vi "Process.vi"(8 "error in":errorcluster, 11 "Plugin in":refnum<class "DFT_Spectra.lvclass">) -> (0 "error out":errorcluster, 3 "Plugin out":refnum<class "DFT_Spectra.lvclass">)   [LabVIEW 2024, in "DFT_Spectra.lvlib" / "DFT_Spectra.lvclass"]
uses:
  DFT_Spectra.lvclass
  DFT_Spectra.lvclass/DFT_Spectra.ctl
  <vilib>/addons/_NISVFA/_Shared subVIs/Data Objects/Waveforms (DBL)/SV Read Next Overlapping Data.vi
  <vilib>/FlexLogger/SDK/PluginSDK.lvlibp/PEFClasses/SDK/Plugin/Plugin.lvclass
  <vilib>/addons/_NISVFA/_Shared subVIs/Data Objects/Waveforms (DBL)/Waveforms (N Ch).lvclass
  C:/Program Files/National Instruments/LabVIEW 2024/vi.lib/FlexLogger/SDK/PluginSDK.lvlibp/PEFClasses/SDK/Plugin/Plugin.lvclass
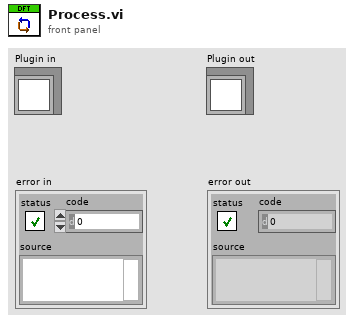
[diagram p1: front panel]
types:
  T1 = typedef "DFT_Spectra.lvlib/DFT_Spectra.lvclass/DFT_Spectra Data.ctl" = cluster{"First Time":bool, "Show Results Window":bool, "Show Results Window Clicked":bool, "Window":T2, "overlap":i32, "Block Duration":dbl, "Averaging parameters":cluster{"averaging mode":enum16{"No averaging", "Vector averaging", "RMS averaging", "Peak hold"}, "weighting mode":enum16{"Linear", "Exponential"}, "number of averages":u32}, "buffer out":refnum<data-value>, "Avg Spectra":refnum<vi>, "Spectra UI":refnum<vi>}
  T2 = typedef "NI_AALPro.lvlib/windowTd.ctl" = u32
  T3 = typedef "svc_Spectrum Info.ctl" = cluster{"channel name":string, "description":string, "x-axis units":T4, "spectral info":cluster{"spectrum type":T5, "linear/dB":enum16{"linear", "dB"}, "window":u16, "window size":i32, "FFT size":i32}, "engineering units":T6, "custom label":string, "dB reference [EU]":dbl, "peak units":enum16{"rms", "peak", "peak-peak"}, "weighting filter":T7, "spectral density?":bool, "unit label":string, "spectrum skewed?":bool, "complimentary spectrum units":T8}
  T4 = typedef "svc_X-Axis Units.ctl" = u16
  T5 = typedef "svc_Spectrum Type.ctl" = enum16{"FFT Spectrum [complex]", "Amplitude [Magnitude]", "Power [Magnitude^2]", "Cross Spectrum [complex]", "Frequency Response [Complex]"}
  T6 = typedef "svc_Engineering Units Text Ring.ctl" = u16
  T7 = typedef "svc_Weighting Filter Text Ring.ctl" = u16
  T8 = typedef "svc_Complimentary Spectrum Units.ctl" = enum16{"none", "radians", "degrees", "cycles", "imaginary"}
  T9 = cluster{"power spectra":cluster{"f0":dbl, "df":dbl, "magnitude":dbl[]}[], "spectra info":T3[], "data valid":bool, "averages completed":dbl}
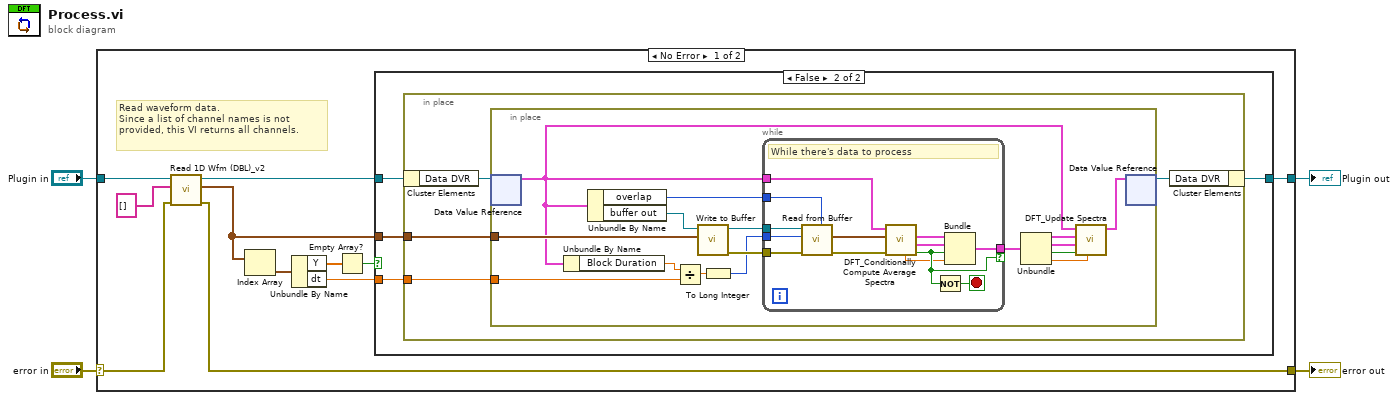
[diagram p0: block diagram]
diagram:
  n1 = case shown="No Error" "error in" {
    selector: "error in" -> [w14 w54]
    tunnel: [w13 w55] -> w3
    tunnel: "Plugin in" -> [w15 w55]
    tunnel: [w5 w54] -> w2
    frame No Error {
      # "Read waveform data.\nSince a list of channel names is not provided, this VI returns all channels."
      n2 = call <vilib>:"Read 1D Wfm (DBL)_v2.vi"("error in (no error)"=w14, "Unique Identifers (empty = all)"=string[] [] ("Unique Channel Identifers (empty = all)"), "Plugin in"=w15) -> ("error out"=w5:errorcluster, "Data"=w10:waveform(dbl)[], "Plugin out"=w12:refnum<class "DFT_Spectra.lvclass">)  [unwired: 5 in, 1 out]
      n3 = Index Array(array=w10) -> (element=w9:waveform(dbl))  [unwired: 1 in]
      n4 = Unbundle By Name(w9) -> ("Y"=w8:dbl[], "dt"=w6:dbl)
      n5 = Empty Array?(array=w8) -> (empty?=w7:bool)
      n6 = case shown="False" w7 {
        tunnel: w10 -> [_ w20]
        tunnel: [w16 w17] -> w13
        tunnel: w12 -> [w16 w18]
        tunnel: w6 -> [_ w19]
        frame True {
          # "No channels sending data to the plugin"
        }
        frame False {
          n7 = in-place {
            in-place-border: w20 -> [w24]
            in-place-border: w19 -> [w23]
            n8 = in-place-cluster #1(w18) -> ("Data DVR"=w22:refnum<data-value>)
            n9 = in-place {
              in-place-border: w24 -> [w38]
              in-place-border: w23 -> [w35]
              n10 = in-place-dvr #2(w22) -> (w30:T1)  [unwired: 1 out]
              n11 = Unbundle By Name(w30) -> ("Block Duration"=w34:dbl)
              n12 = Unbundle By Name(w30) -> ("overlap"=w31:i32, "buffer out"=w39:refnum<data-value>)
              n13 = Divide(x=w34, y=w35) -> (x/y=w33:dbl)
              n14 = call <vilib>:"Write to Buffer.vi"("waveforms"=w38, "buffer"=w39) -> ("error out"=w36:errorcluster, "buffer out"=w37:refnum<data-value>)  [unwired: 7 in, 1 out]
              n15 = To Long Integer(number=w33) -> (32bit integer=w32:i32)
              n16 = while {
                tunnel: w37 -> [w53]
                tunnel: w36 -> [w52]
                tunnel: w32 -> [w51]
                tunnel: w31 -> [w50]
                tunnel: [w41] -> w29 if=w43
                tunnel: w30 -> [w46]
                stop <- w48 stop-if-true
                # "While there's data to process"
                n17 = call-poly <vilib>:"Read from Buffer.vi"("overlap (50 %)"=w50, "error in (no error)"=w52, "block length (4096 samples)"=w51, "buffer"=w53) -> ("error out"=w49:errorcluster, "waveforms subset"=w47:waveform(dbl)[])  [unwired: 4 in, 2 out]
                n18 = call "DFT_Conditionally Compute Average Spectra.vi"("error in"=w49, "waveforms subset"=w47, "Data"=w46) -> ("data valid"=w43:bool, "spectra info"=w44:T3[], "power spectra"=w45:cluster{"f0":dbl, "df":dbl, "magnitude":dbl[]}[], "averages completed"=w42:dbl)  [unwired: 5 in]
                n19 = Not(x=w43) -> (.not. x?=w48:bool)
                n20 = Bundle("power spectra"=w45, "spectra info"=w44, "data valid"=w43, "averages completed"=w42) -> (w41:T9)  [unwired: 1 in]
              }
              n21 = Unbundle(w29) -> ("power spectra"=w27:cluster{"f0":dbl, "df":dbl, "magnitude":dbl[]}[], "spectra info"=w26:T3[], "data valid"=w25:bool, "averages completed"=w28:dbl)
              n22 = call "DFT_Update Spectra.vi"("averages completed"=w28, "data valid"=w25, "spectra info"=w26, "spectra"=w27, "Data"=w30) -> ("Data out"=w40:T1)  [unwired: 6 in]
              n23 = in-place-dvr #2(w40) -> (w21:refnum<data-value>)  [unwired: 1 out]
            }
            n24 = in-place-cluster #1("Data DVR"=w21) -> (w17:refnum<class "DFT_Spectra.lvclass">)
          }
        }
      }
    }
    frame Error {
    }
  }
  "error out" <- w2
  "Plugin out" <- w3
